vi "UHR-Fleezers Control (host) - 11.8.vi"() -> ()   [LabVIEW 2014] (continued)
                n1966 = property on="Sample Channel\nFlow" class="Bool (strict)"("Val(Sgnl)"=TRUE ("Value (Signaling)")) -> ()  [unwired: 2 in, 2 out]
              }
            }
          }
          frame #1 {
            n1967 = property on="Inject Pump 3" class="Bool (strict)"("Val(Sgnl)"=FALSE ("Value (Signaling)")) -> ()  [unwired: 2 in, 2 out]
            n1968 = local write "Target"(FALSE ("Target")) -> ()
          }
          frame #2 {
            n1969 = property on="Move Cap. 1 (DNA Bottom)" class="Bool (strict)"("Val(Sgnl)"=TRUE ("Value (Signaling)")) -> ()  [unwired: 2 in, 2 out]
          }
        }
      }
      event "Force FB Script": Value Change {
        n1970 = event-data() -> ()  [unwired: 1 in, 5 out]
        n1971 = local write "Force FB Script"(FALSE ("Force FB Data\nScript")) -> ()
        n1972 = flat-sequence {
          tunnel: w2821 -> [w2825]
          tunnel: w2822 -> [w2826]
          tunnel: [w2826] -> w2817
          tunnel: [w2825] -> w2816
          tunnel: w2817 -> [w2829]
          tunnel: w2816 -> [w2828]
          tunnel: ["Trap Trig Fl."] -> w2818
          tunnel: [w2871] -> w2819
          tunnel: w2818 -> [w2871]
          tunnel: [w2875] -> w2820
          tunnel: w2819 -> [w2875]
          tunnel: w2820 -> [w2877]
          frame #0 {
            n1973 = property on="Trap D (MHz)" class="DigNum (strict)"("Val(Sgnl)"="Trap D Before Moving") -> ()  [unwired: 2 in, 2 out]
          }
          frame #1 {
            n1974 = local read "Saved Stage Positions"() -> (w2831:dbl[][])
            n1975 = local write "FB Trap Pos Offset"(0.0 ("FB Trap Pos Offset")) -> ()
            n1976 = property on="Trap Pos. FB Offset Factor" class="DigNum (strict)"("Val(Sgnl)"=i64 0 ("Value (Signaling)")) -> ()  [unwired: 2 in, 2 out]
            n1977 = local write "Stage Moving"(TRUE ("Stage Moving")) -> ()
            n1978 = call "move to saved stage position.vi"("error in"=w2828, "Stage VISA resource name in"=w2829, "Position"="Stage Position To Establish FB", "Saved Stage Positions"=w2831) -> ("error out"=w2827:errorcluster)  [unwired: 1 out]
            n1979 = local write "Stage Control Serial Error"(w2827) -> ()
          }
          frame #2 {
            n1980 = call <vilib>:"Beep.vi"("duration (msec)"=u32 100, "frequency (Hz)"=u32 20) -> ()  [unwired: 1 in, 9 out]
            n1981 = local write "Stage Moving"(FALSE ("Stage Moving")) -> ()
            n1982 = property on="Tab Control 2" class="TabCtl (strict)"("Val(Sgnl)"=T6."Feedback on Trap Position" ("Value (Signaling)")) -> ()  [unwired: 2 in, 2 out]
            n1983 = stacked-sequence {
              frame #0 {
                n1984 = Multiply(x="Wait (s)", y=u32 1000 ("milliseconds to wait")) -> (x*y=w2840:u32)
                n1985 = property on="Trap D (MHz)" class="DigNum (strict)"("Val(Sgnl)"="Starting Trap D (MHz)") -> ()  [unwired: 2 in, 2 out]
                n1986 = Wait (ms)(milliseconds to wait=w2840) -> ()  [unwired: 1 out]
              }
              frame #1 {
                n1987 = property on="Set Reading to\nSetpoint" class="Bool (strict)"("Val(Sgnl)"=TRUE ("Value (Signaling)")) -> ()  [unwired: 2 in, 2 out]
              }
            }
            n1988 = property on="Tab Control" class="TabCtl (strict)"("Val(Sgnl)"=T4."Trap Control (RF)" ("Value (Signaling)")) -> ()  [unwired: 2 in, 2 out]
          }
          frame #3 {
            n1989 = Wait (ms)(milliseconds to wait=u32 500) -> ()  [unwired: 1 out]
          }
          frame #4 {
            n1990 = property on="Trap Pos. FB ON" class="Bool (strict)"("Val(Sgnl)"=TRUE ("Value (Signaling)")) -> ()  [unwired: 2 in, 2 out]
            n1991 = Wait (ms)(milliseconds to wait=u32 250) -> ()  [unwired: 1 out]
          }
          frame #5 {
            n1992 = case shown="\"0\", Default" "Remove Action Offset Dropdown" {
              tunnel: TRUE ("Value (Signaling)") -> [w2852 w2860 w2868]
              frame "1" {
                n1993 = flat-sequence {
                  tunnel: w2852 -> [w2859]
                  frame #0 {
                    n1994 = local read "factor"() -> (w2854:dbl)
                    n1995 = Greater Than 0?(x=w2854) -> (x > 0?=w2858:bool)
                    n1996 = Select(t=1.0, s=w2858, f=-1.0) -> (s? t:f=w2855:dbl)
                    n1997 = Multiply(x=w2855, y=w2854) -> (x*y=w2853:dbl)
                    n1998 = local write "factor"(w2853) -> ()
                  }
                  frame #1 {
                    n1999 = property on="Remove Offset to factor" class="Bool (strict)"("Val(Sgnl)"=w2859) -> ()  [unwired: 2 in, 2 out]
                  }
                }
              }
              frame "2" {
                n2000 = flat-sequence {
                  tunnel: w2860 -> [w2867]
                  frame #0 {
                    n2001 = local read "factor"() -> (w2861:dbl)
                    n2002 = Greater Than 0?(x=w2861) -> (x > 0?=w2866:bool)
                    n2003 = Select(t=-1.0, s=w2866, f=1.0) -> (s? t:f=w2864:dbl)
                    n2004 = Multiply(x=w2861, y=w2864) -> (x*y=w2863:dbl)
                    n2005 = local write "factor"(w2863) -> ()
                  }
                  frame #1 {
                    n2006 = property on="Remove Offset to factor" class="Bool (strict)"("Val(Sgnl)"=w2867) -> ()  [unwired: 2 in, 2 out]
                  }
                }
              }
              frame "0", Default {
                n2007 = property on="Remove Action Offset" class="Bool (strict)"("Val(Sgnl)"=w2868) -> ()  [unwired: 2 in, 2 out]
              }
            }
            n2008 = case shown="False" "Trap Trig Fl." {
              frame False {
                n2009 = case shown="True" "Green ON after FB ON?" {
                  selector: "Green ON after FB ON?" -> [_ w2870]
                  frame False {
                  }
                  frame True {
                    n2010 = property on="Green Laser ON/Interlacing" class="Bool (strict)"("Val(Sgnl)"=w2870) -> ()  [unwired: 2 in, 2 out]
                  }
                }
              }
              frame True {
              }
            }
            n2011 = Wait (ms)(milliseconds to wait=u32 250) -> ()  [unwired: 1 out]
          }
          frame #6 {
            n2012 = property on="Start Saving" class="Bool (strict)"("Val(Sgnl)"=TRUE ("Value (Signaling)")) -> ()  [unwired: 2 in, 2 out]
            n2013 = Wait (ms)(milliseconds to wait=u32 5000) -> ()  [unwired: 1 out]
          }
          frame #7 {
            w2874 = TRUE ("Value (Signaling)")
            n2014 = property on="Rem fb disp offset" class="Bool (strict)"("Val(Sgnl)"=w2874) -> ()  [unwired: 2 in, 2 out]
            n2015 = property on="Remove Offset" class="Bool (strict)"("Val(Sgnl)"=w2874) -> ()  [unwired: 2 in, 2 out]
            n2016 = Wait (ms)(milliseconds to wait=u32 100) -> ()  [unwired: 1 out]
          }
          frame #8 {
            n2017 = case shown="True" w2877 {
              frame False {
              }
              frame True {
                n2018 = local write "Trap Trig. Fl."(TRUE ("Value (Signaling)")) -> ()
              }
            }
          }
          frame #9 {
            n2019 = local read "Tether"() -> (w2880:bool)
            n2020 = And(x="Start dipping after?", y=w2880) -> (x .and. y?=w2879:bool)
            n2021 = case shown="True" w2879 {
              frame False {
              }
              frame True {
                n2022 = flat-sequence {
                  frame #0 {
                    n2023 = Multiply(x="Delay before dipping (s)", y=1000.0) -> (x*y=w2883:dbl)
                    n2024 = Wait (ms)(milliseconds to wait=w2883) -> ()  [unwired: 1 out]
                  }
                  frame #1 {
                    n2025 = property on="Dip for Protein" class="Bool (strict)"("Val(Sgnl)"=TRUE ("Value (Signaling)")) -> ()  [unwired: 2 in, 2 out]
                    n2026 = local write "Scripts"(T29."Dipping") -> ()
                  }
                }
              }
            }
          }
        }
      }
      event "Rupture Script": Value Change {
        n2027 = event-data() -> ()  [unwired: 1 in, 5 out]
        n2028 = local write "Rupture Script"(FALSE ("Rupture Script")) -> ()
        n2029 = flat-sequence {
          frame #0 {
            w2889 = TRUE
            w2894 = FALSE
            # "Number 6 for now is the\nrupture-experiment\nparameters."
            n2030 = local read "Starting Trap D (MHz)"() -> (w2895:dbl)
            n2031 = local write "Restart DMA? (AOD)"(w2894) -> ()
            n2032 = Replace Array Subset(array=u32[] [0] ("Index Values"), new element=6, index=0) -> (w2890:u32[])
            n2033 = local write "Save scans"(w2894) -> ()
            n2034 = property on="Trap D (MHz)" class="DigNum (strict)"("Val(Sgnl)"=w2895) -> ()  [unwired: 2 in, 2 out]
            n2035 = property on="Saved AOD Raster Scan Parameter Sets" class="Arr (strict)"("Index Values"=w2890) -> ()  [unwired: 2 in, 2 out]
            n2036 = property on="Start Saving" class="Bool (strict)"("Val(Sgnl)"=w2889) -> ()  [unwired: 2 in, 2 out]
            n2037 = property on="Green Laser ON/Interlacing" class="Bool (strict)"("Val(Sgnl)"=w2889) -> ()  [unwired: 2 in, 2 out]
          }
          frame #1 {
            n2038 = property on="Load parameters" class="Bool (strict)"("Val(Sgnl)"=TRUE ("Value (Signaling)")) -> ()  [unwired: 2 in, 2 out]
          }
        }
      }
      event "Fixed Traps Script": Value Change {
        n2039 = event-data() -> ()  [unwired: 1 in, 5 out]
        n2040 = local write "Fixed Traps Script"(FALSE ("Fixed Traps Data\nScript")) -> ()
        n2041 = flat-sequence {
          frame #0 {
            n2042 = case shown="True" "Green ON" {
              frame False {
              }
              frame True {
                n2043 = property on="Green Laser ON/Interlacing" class="Bool (strict)"("Val(Sgnl)"=TRUE) -> ()  [unwired: 2 in, 2 out]
              }
            }
            n2044 = local write "Offset (nm)"(0.0 ("Offset (nm)")) -> ()
            n2045 = property on="Sample Channel\nFlow" class="Bool (strict)"("Val(Sgnl)"=FALSE ("Value (Signaling)")) -> ()  [unwired: 2 in, 2 out]
            n2046 = property on="Trap D (MHz)" class="DigNum (strict)"("Val(Sgnl)"="Fixed Traps Trap Delta (MHz)") -> ()  [unwired: 2 in, 2 out]
          }
          frame #1 {
            n2047 = Wait (ms)(milliseconds to wait=u32 1000) -> ()  [unwired: 1 out]
          }
          frame #2 {
            n2048 = local write "Start Saving"(TRUE ("Start Saving")) -> ()
          }
          frame #3 {
            n2049 = local read "Bead Sep. Int. Time (s)"() -> (w2905:dbl)
            n2050 = Multiply(x=w2905, y=1000.0) -> (x*y=w2907:dbl)
            n2051 = Wait (ms)(milliseconds to wait=w2907) -> ()  [unwired: 1 out]
          }
          frame #4 {
            n2052 = property on="Remove Offset" class="Bool (strict)"("Val(Sgnl)"=TRUE ("Value (Signaling)")) -> ()  [unwired: 2 in, 2 out]
          }
          frame #5 {
            n2053 = property on="Dip for Protein" class="Bool (strict)"("Val(Sgnl)"="Start dipping after?") -> ()  [unwired: 2 in, 2 out]
          }
        }
      }
      event "Got DNA bead": Value Change {
        n2054 = event-data() -> ()  [unwired: 1 in, 5 out]
        n2055 = flat-sequence {
          frame #0 {
            n2056 = local read "Daq spot flow on"() -> (w2912:bool)
            n2057 = case shown="True" w2912 {
              frame False {
              }
              frame True {
                n2058 = property on="Sample Channel\nFlow" class="Bool (strict)"("Val(Sgnl)"=TRUE ("Value (Signaling)")) -> ()  [unwired: 2 in, 2 out]
              }
            }
            n2059 = property on="Got DNA bead" class="Bool"("Key Focus"=FALSE) -> ()  [unwired: 2 in, 2 out]
          }
          frame #1 {
            n2060 = property on="Inject Pump 1" class="Bool (strict)"("Val(Sgnl)"=FALSE ("Value (Signaling)")) -> ()  [unwired: 2 in, 2 out]
          }
          frame #2 {
            n2061 = property on="Cal/Data Acq. Spot" class="Bool (strict)"("Val(Sgnl)"=TRUE ("Value (Signaling)")) -> ()  [unwired: 2 in, 2 out]
          }
        }
      }
      event "Take Stepping Data": Value Change {
        n2062 = event-data() -> ()  [unwired: 1 in, 5 out]
        n2063 = local read "Save ave N"() -> (w2924:dbl)
        n2064 = flat-sequence {
          tunnel: w2924 -> [w2926]
          tunnel: [w2926] -> w2919
          tunnel: [w2928] -> w2920
          tunnel: w2919 -> [w2928]
          tunnel: [w2930] -> w2921
          tunnel: w2920 -> [w2930]
          tunnel: [w2933] -> w2922
          tunnel: w2921 -> [w2933]
          tunnel: [w2935] -> w2923
          tunnel: w2922 -> [w2935]
          tunnel: [w2937] -> w2917
          tunnel: w2923 -> [w2937]
          tunnel: w2917 -> [w2940]
          tunnel: [w2940] -> w2916
          tunnel: w2916 -> [w2941]
          tunnel: [w2941] -> w2918
          tunnel: w2918 -> [w2947]
          frame #0 {
            n2065 = property on="Save ave N" class="DigNum (strict)"("Val(Sgnl)"="Save ave factor") -> ()  [unwired: 2 in, 2 out]
          }
          frame #1 {
            n2066 = Wait (ms)(milliseconds to wait=u32 100) -> ()  [unwired: 1 out]
          }
          frame #2 {
            n2067 = local read "Offset 2 Start (MHz)"() -> (w2932:dbl)
            n2068 = property on="Saved AOD Raster Scan Parameter Sets" class="Arr (strict)"("Index Values"=u32[] [2]) -> ()  [unwired: 2 in, 2 out]
            n2069 = property on="Trap D (MHz)" class="DigNum (strict)"("Val(Sgnl)"=w2932) -> ()  [unwired: 2 in, 2 out]
          }
          frame #3 {
            n2070 = property on="Load parameters" class="Bool (strict)"("Val(Sgnl)"=TRUE ("Value (Signaling)")) -> ()  [unwired: 2 in, 2 out]
          }
          frame #4 {
            n2071 = Wait (ms)(milliseconds to wait=u32 100) -> ()  [unwired: 1 out]
          }
          frame #5 {
            n2072 = property on="Trap Raster Scan" class="Bool (strict)"("Val(Sgnl)"=TRUE ("Value (Signaling)")) -> ()  [unwired: 2 in, 2 out]
          }
          frame #6 {
            n2073 = Wait (ms)(milliseconds to wait=u32 1000) -> ()  [unwired: 1 out]
          }
          frame #7 {
            n2074 = while {
              stop <- w2944 stop-if-true
              n2075 = local read "Raster Scanning..."() -> (w2946:bool)
              n2076 = local read "Saving..."() -> (w2945:bool)
              n2077 = Not(x=w2945) -> (.not. x?=w2942:bool)
              n2078 = Not(x=w2946) -> (.not. x?=w2943:bool)
              n2079 = And(x=w2943, y=w2942) -> (x .and. y?=w2944:bool)
            }
          }
          frame #8 {
            n2080 = property on="Save ave N" class="DigNum (strict)"("Val(Sgnl)"=w2947) -> ()  [unwired: 2 in, 2 out]
          }
        }
      }
      event "Step Size (nm)": Value Change {
        n2081 = event-data() -> ()  [unwired: 1 in, 5 out]
        n2082 = flat-sequence {
          frame #0 {
            n2083 = property on="Saved AOD Raster Scan Parameter Sets" class="Arr (strict)"("Index Values"=u32[] [1]) -> ()  [unwired: 2 in, 2 out]
          }
          frame #1 {
            n2084 = Multiply(x="N Steps", y="Step Size (nm)") -> (x*y=w2949:dbl)
            n2085 = property on="Scan Speed AOD (nm/s) 2" class="DigNum (strict)"("Value"="Step Size (nm)") -> ()  [unwired: 2 in, 2 out]
            n2086 = property on="Step Size AOD (nm) 2" class="DigNum (strict)"("Value"="Step Size (nm)") -> ()  [unwired: 2 in, 2 out]
            n2087 = property on="Scan Range AOD (nm) 2" class="DigNum (strict)"("Value"=w2949) -> ()  [unwired: 2 in, 2 out]
          }
        }
      }
      event "Take Detection Laser\nImage": Value Change {
        n2088 = event-data() -> ()  [unwired: 1 in, 5 out]
        n2089 = flat-sequence {
          tunnel: [w2977] -> w2967
          tunnel: [w2976] -> w2960
          tunnel: [w2975] -> w2952
          tunnel: [w2980] -> w2968
          tunnel: w2967 -> [w2980]
          tunnel: [w2979] -> w2961
          tunnel: w2960 -> [w2979]
          tunnel: [w2978] -> w2953
          tunnel: w2952 -> [w2978]
          tunnel: [w2984] -> w2969
          tunnel: w2968 -> [w2984]
          tunnel: [w2983] -> w2962
          tunnel: w2961 -> [w2983]
          tunnel: [w2982] -> w2954
          tunnel: w2953 -> [w2982]
          tunnel: [w2990] -> w2970
          tunnel: w2969 -> [w2990]
          tunnel: [w2989] -> w2963
          tunnel: w2962 -> [w2989]
          tunnel: [w2988] -> w2955
          tunnel: w2954 -> [w2988]
          tunnel: [w2994] -> w2971
          tunnel: w2970 -> [w2994]
          tunnel: [w2993] -> w2964
          tunnel: w2963 -> [w2993]
          tunnel: [w2992] -> w2956
          tunnel: w2955 -> [w2992]
          tunnel: [w2998] -> w2972
          tunnel: w2971 -> [w2998]
          tunnel: [w2997] -> w2965
          tunnel: w2964 -> [w2997]
          tunnel: [w2996] -> w2957
          tunnel: w2956 -> [w2996]
          tunnel: [w3002] -> w2973
          tunnel: w2972 -> [w3002]
          tunnel: [w3001] -> w2966
          tunnel: w2965 -> [w3001]
          tunnel: [w3000] -> w2958
          tunnel: w2957 -> [w3000]
          tunnel: w2973 -> [w3008]
          tunnel: w2966 -> [w3007]
          tunnel: [w3005] -> w2959
          tunnel: w2958 -> [w3005]
          tunnel: w2959 -> [w3009]
          frame #0 {
            n2090 = local read "Green Laser ON/Interlacing"() -> (w2977:bool)
            n2091 = local read "Green laser mode"() -> (w2976:enum32{"Laser ON", "Laser OFF", "Interlace"})
            n2092 = local read "Green FB On/Off"() -> (w2975:bool)
          }
          frame #1 {
            n2093 = property on="Green FB On/Off" class="Bool (strict)"("Val(Sgnl)"=FALSE ("Value (Signaling)")) -> ()  [unwired: 2 in, 2 out]
          }
          frame #2 {
            n2094 = property on="Green Laser ON/Interlacing" class="Bool (strict)"("Val(Sgnl)"=TRUE ("Value (Signaling)")) -> ()  [unwired: 2 in, 2 out]
            n2095 = property on="Flip Green Filter" class="Bool (strict)"("Val(Sgnl)"=TRUE ("Value (Signaling)")) -> ()  [unwired: 2 in, 2 out]
            n2096 = property on="Green laser mode" class="RadioBtnsControl (strict)"("Val(Sgnl)"=enum32{"Laser ON", "Laser OFF", "Interlace"}."Laser ON" ("Value (Signaling)")) -> ()  [unwired: 2 in, 2 out]
          }
          frame #3 {
            n2097 = Wait (ms)(milliseconds to wait=u32 500) -> ()  [unwired: 1 out]
          }
          frame #4 {
            n2098 = property on="Confocal\nImage" class="Bool (strict)"("Val(Sgnl)"=TRUE ("Value (Signaling)")) -> ()  [unwired: 2 in, 2 out]
          }
          frame #5 {
            n2099 = Wait (ms)(milliseconds to wait=u32 2000) -> ()  [unwired: 1 out]
          }
          frame #6 {
            n2100 = while {
              stop <- w3003 stop-if-true
              n2101 = local read "Saving..."() -> (w3004:bool)
              n2102 = Not(x=w3004) -> (.not. x?=w3003:bool)
            }
          }
          frame #7 {
            n2103 = property on="Flip Green Filter" class="Bool (strict)"("Val(Sgnl)"=TRUE ("Value (Signaling)")) -> ()  [unwired: 2 in, 2 out]
            n2104 = property on="Green Laser ON/Interlacing" class="Bool (strict)"("Val(Sgnl)"=w3008) -> ()  [unwired: 2 in, 2 out]
            n2105 = property on="Green laser mode" class="RadioBtnsControl (strict)"("Val(Sgnl)"=w3007) -> ()  [unwired: 2 in, 2 out]
          }
          frame #8 {
            n2106 = property on="Green FB On/Off" class="Bool (strict)"("Val(Sgnl)"=w3009) -> ()  [unwired: 2 in, 2 out]
          }
        }
      }
      event "Stop All": Value Change {
        n2107 = event-data() -> ()  [unwired: 1 in, 5 out]
        n2108 = local read "Stop All"() -> (w3010:bool)
      }
    }
    n2109 = node-c288() -> ()  [unwired: 1 in, 1 out]
  }
  n2110 = timed-loop "Mouse control: trap position (AOM deflection), set confocal spot from image" {
    tunnel: [w3012] -> w198
    tunnel: w18 -> [w3011]
    timing: w110 -> [_]
    timing-out: [_] -> w109
    stop <- w3012 stop-if-true
    n2111 = node-c288() -> ()  [unwired: 2 out]
    n2112 = event shown="[0] \"Pane\": Mouse Down" {
      selector: _ -> [_ _]
      dyn-events: _ -> [_ _]
      timeout: _ -> [_ _]
      tunnel: w3011 -> [w3015 _]
      event Mouse Down {
        n2113 = event-data() -> ("Time"=w3017:u32, "Coords"=w3016:T7, "Button"=w3018:u16)  [unwired: 6 out]
        n2114 = case shown="3" w3018 {
          tunnel: w3017 -> [_ _ w3157]
          tunnel: w3016 -> [_ w3023 w3155]
          tunnel: w3015 -> [_ _ w3153]
          frame 0, Default {
          }
          frame 1 {
            n2115 = property on="APD 2" class="ImageControl"() -> ("Displayed Image Position"=w3037:cluster{"Left":i32, "Top":i32})  [unwired: 2 in, 2 out]
            n2116 = control-ref of="Primary Video Display"() -> (w3030:refnum<vi>)
            n2117 = property on="APD 1" class="ImageControl"() -> ("Displayed Image Position"=w3066:cluster{"Left":i32, "Top":i32})  [unwired: 2 in, 2 out]
            n2118 = property on="Detection Laser X" class="ImageControl"() -> ("Displayed Image Position"=w3063:cluster{"Left":i32, "Top":i32})  [unwired: 2 in, 2 out]
            n2119 = property on="Detection Laser Y" class="ImageControl"() -> ("Displayed Image Position"=w3062:cluster{"Left":i32, "Top":i32})  [unwired: 2 in, 2 out]
            n2120 = property on="APD 2" class="ImageControl"() -> ("Displayed Image Size"=w3036:cluster{"Width":u32, "Height":u32})  [unwired: 2 in, 2 out]
            n2121 = property on="APD 1" class="ImageControl"() -> ("Displayed Image Size"=w3064:cluster{"Width":u32, "Height":u32})  [unwired: 2 in, 2 out]
            n2122 = property on="Detection Laser X" class="ImageControl"() -> ("Displayed Image Size"=w3065:cluster{"Width":u32, "Height":u32})  [unwired: 2 in, 2 out]
            n2123 = property on="Detection Laser Y" class="ImageControl"() -> ("Displayed Image Size"=w3061:cluster{"Width":u32, "Height":u32})  [unwired: 2 in, 2 out]
            n2124 = property class="ImageControl"(reference=w3030) -> ("Displayed Image Position"=w3028:cluster{"Left":i32, "Top":i32})  [unwired: 1 in, 2 out]
            n2125 = property class="ImageControl"(reference=w3030) -> ("Displayed Image Size"=w3029:cluster{"Width":u32, "Height":u32})  [unwired: 1 in, 2 out]
            n2126 = Unbundle By Name(w3036) -> ("Width"=w3033:u32, "Height"=w3032:u32)
            n2127 = Unbundle By Name(w3037) -> ("Left"=w3035:i32, "Top"=w3034:i32)
            n2128 = Unbundle By Name(w3064) -> ("Width"=w3058:u32, "Height"=w3057:u32)
            n2129 = Unbundle By Name(w3065) -> ("Width"=w3054:u32, "Height"=w3053:u32)
            n2130 = Unbundle By Name(w3061) -> ("Width"=w3050:u32, "Height"=w3049:u32)
            n2131 = Unbundle By Name(w3066) -> ("Left"=w3060:i32, "Top"=w3059:i32)
            n2132 = Unbundle By Name(w3063) -> ("Left"=w3056:i32, "Top"=w3055:i32)
            n2133 = Unbundle By Name(w3062) -> ("Left"=w3052:i32, "Top"=w3051:i32)
            n2134 = Bundle("Left"=w3035, "Top"=w3034, "Width"=w3033, "Height"=w3032) -> (w3031:T30)  [unwired: 1 in]
            n2135 = Bundle("Left"=w3060, "Top"=w3059, "Width"=w3058, "Height"=w3057) -> (w3048:T30)  [unwired: 1 in]
            n2136 = Bundle("Left"=w3056, "Top"=w3055, "Width"=w3054, "Height"=w3053) -> (w3047:T30)  [unwired: 1 in]
            n2137 = Bundle("Left"=w3052, "Top"=w3051, "Width"=w3050, "Height"=w3049) -> (w3046:T30)  [unwired: 1 in]
            n2138 = Unbundle By Name(w3029) -> ("Width"=w3025:u32, "Height"=w3024:u32)
            n2139 = Unbundle By Name(w3028) -> ("Left"=w3027:i32, "Top"=w3026:i32)
            n2140 = Build Cluster Array(w3031, w3048, w3047, w3046) -> (w3045:T31)
            n2141 = Bundle("Left"=w3027, "Top"=w3026, "Width"=w3025, "Height"=w3024) -> (w3020:T30)  [unwired: 1 in]
            n2142 = for {
              tunnel: w3023 -> [w3099]
              tunnel: w3045 -> [w3100] mode=indexing
              shift-right: [w3097] -> w3043
              shift-left: TRUE -> [w3098]
              shift-right: [w3096] -> w3041
              shift-left: _ -> [w3092]
              shift-right: [w3095] -> w3040
              shift-left: _ -> [w3091]
              shift-right: [w3094] -> w3039
              shift-left: _ -> [w3090]
              shift-right: [w3093] -> w3038
              shift-left: _ -> [w3089]
              n2143 = case shown="True" w3098 {
                selector: w3098 -> [w3105 _]
                tunnel: w3100 -> [_ w3114]
                tunnel: w3099 -> [_ w3112]
                tunnel: [w3105 w3110] -> w3097
                tunnel: [w3104 w3109] -> w3096
                tunnel: [w3103 w3108] -> w3095
                tunnel: [w3102 w3107] -> w3094
                tunnel: [w3101 w3106] -> w3093
                tunnel: w3092 -> [w3104 _]
                tunnel: w3091 -> [w3103 _]
                tunnel: w3090 -> [w3102 _]
                tunnel: w3089 -> [w3101 _]
                frame False {
                }
                frame True {
                  n2144 = Unbundle(w3114) -> (w3113:T30)
                  n2145 = call "isclickinwindow.vi"("Image Param"=w3113, "Point32"=w3112) -> ("4 Y"=w3106:i32, "3 Height"=w3107:i32, "2 X"=w3108:i32, "1 Width"=w3109:i32, "In image?"=w3111:bool)  [unwired: 1 in]
                  n2146 = Not(x=w3111) -> (.not. x?=w3110:bool)
                }
              }
            }
            n2147 = call "isclickinwindow.vi"("Image Param"=w3020, "Point32"=w3023) -> ("4 Y"=w3021:i32, "2 X"=w3022:i32, "In image?"=w3019:bool)  [unwired: 1 in, 2 out]
            n2148 = case shown="True" w3019 {
              tunnel: w3022 -> [_ w3070]
              tunnel: w3021 -> [_ w3073]
              frame False {
              }
              frame True {
                w3082 = 2
                n2149 = Subtract(x=480, y=w3073) -> (x-y=w3072:i32)
                n2150 = Unbundle("Target size") -> ("Width"=w3083:dbl, "Height"=w3081:dbl)
                n2151 = Subtract(x=w3070, y=2) -> (x-y=w3069:i32)
                n2152 = Divide(x=w3081, y=w3082) -> (x/y=w3079:dbl)
                n2153 = Divide(x=w3083, y=w3082) -> (x/y=w3080:dbl)
                n2154 = Subtract(x=w3069, y=w3080) -> (x-y=w3078:dbl)
                n2155 = Add(x=w3069, y=w3080) -> (x+y=w3076:dbl)
                n2156 = Subtract(x=w3072, y=w3079) -> (x-y=w3077:dbl)
                n2157 = Add(x=w3072, y=w3079) -> (x+y=w3075:dbl)
                n2158 = Bundle(w3069, w3072) -> (w3085:cluster{i32, i32})  [unwired: 1 in]
                n2159 = Bundle(w3078, w3077, w3076, w3075) -> (w3067:cluster{dbl, dbl, dbl, dbl})  [unwired: 1 in]
                n2160 = case shown="True" "Set target" {
                  tunnel: w3085 -> [_ w3088]
                  tunnel: w3067 -> [_ w3086]
                  frame False {
                  }
                  frame True {
                    n2161 = local write "Target coordinates"(w3086) -> ()
                    n2162 = local write "Set target"(FALSE ("Set target")) -> ()
                    "Video coordinates" <- w3088
                  }
                }
              }
            }
            n2163 = Not(x=w3043) -> (.not. x?=w3042:bool)
            n2164 = case shown="True" w3042 {
              tunnel: w3040 -> [_ w3128]
              tunnel: w3038 -> [_ w3127]
              tunnel: w3041 -> [_ w3126]
              tunnel: w3039 -> [_ w3125]
              frame False {
              }
              frame True {
                w3115 = FALSE ("Get Point")
                n2165 = local read "Scan lines (y)"() -> (w3130:u64)
                n2166 = disable-structure shown="Disabled" {
                  frame Disabled {
                  }
                  frame Enabled {
                  }
                }
                n2167 = local read "Actual MCL Inc (V)"() -> (w3124:dbl)
                n2168 = local read "Scan steps (MCL)"() -> (w3129:u64)
                n2169 = Divide "Y Pix/step"(x=w3125, y=w3130) -> (x/y=w3137:dbl)
                n2170 = Divide "Y V/pix"(x=w3124, y=w3137) -> (x/y=w3136:dbl)
                n2171 = Divide "Y half step offset"(x=w3124, y=2.0) -> (x/y=w3138:dbl)
                n2172 = Divide "X pix/step"(x=w3126, y=w3129) -> (x/y=w3135:dbl)
                n2173 = Negate(x=w3138) -> (-x=w3139:dbl)
                n2174 = local read "Initial Y"() -> (w3145:dbl)
                n2175 = Multiply(x=w3127, y=w3136) -> (x*y=w3146:dbl)
                n2176 = Divide "X half step offset"(x=w3124, y=2.0) -> (x/y=w3132:dbl)
                n2177 = Divide "X V/pix"(x=w3124, y=w3135) -> (x/y=w3134:dbl)
                n2178 = Multiply(x=w3124, y=w3129) -> (x*y=w3141:dbl)
                n2179 = Compound Arithmetic op=ADD(w3139, w3146, w3145) -> (w3116:dbl)
                "Pointer Y (V)" <- w3116
                n2180 = Multiply(x=w3134, y=w3128) -> (x*y=w3143:dbl)
                n2181 = Negate(x=w3132) -> (-x=w3131:dbl)
                n2182 = local read "Initial X"() -> (w3144:dbl)
                n2183 = Negate(x=w3143) -> (-x=w3142:dbl)
                n2184 = Compound Arithmetic op=ADD(w3131, w3141, w3144, w3142) -> (w3117:dbl)
                "Pointer X (V)" <- w3117
                n2185 = case shown="True" "Set High F Confocal Spot (X-Y)" {
                  tunnel: w3117 -> [_ w3147]
                  tunnel: w3116 -> [_ w3148]
                  frame False {
                  }
                  frame True {
                    "Confocal Y 2 (V)" <- w3148
                    "Confocal X 2 (V)" <- w3147
                  }
                }
                n2186 = Or(x="Set X Only", y="Set Confocal Spot (X-Y)") -> (x .or. y?=w3120:bool)
                n2187 = Or(x="Set Confocal Spot (X-Y)", y="Set Y Only") -> (x .or. y?=w3119:bool)
                n2188 = case shown="True" w3120 {
                  tunnel: w3117 -> [_ w3149]
                  frame False {
                  }
                  frame True {
                    n2189 = property on="AO2" class="Slide (strict)"("Val(Sgnl)"=w3149) -> ()  [unwired: 2 in, 2 out]
                    "Confocal X 1 (V)" <- w3149
                  }
                }
                n2190 = case shown="True" w3119 {
                  tunnel: w3116 -> [_ w3150]
                  frame False {
                  }
                  frame True {
                    n2191 = property on="AO1" class="Slide (strict)"("Val(Sgnl)"=w3150) -> ()  [unwired: 2 in, 2 out]
                    "Confocal Y 1 (V)" <- w3150
                  }
                }
                n2192 = local write "Set High F Confocal Spot (X-Y)"(w3115) -> ()
                n2193 = local write "Set Confocal Spot (X-Y)"(w3115) -> ()
                n2194 = local write "Set X Only"(w3115) -> ()
                n2195 = local write "Set Y Only"(w3115) -> ()
              }
            }
          }
          frame 3 {
            n2196 = local read "BD 2 Frequency 1 (MHz)"() -> (w3151:dbl)
            n2197 = local read "BD 1 Frequency 1 (MHz)"() -> (w3152:dbl)
            n2198 = local write "Manipulating Trap"(TRUE ("Manipulating Trap")) -> ()
            n2199 = local write "Coords"(T7 {"Horizontal"=0, "Vertical"=0} ("Coords")) -> ()
            n2200 = while {
              tunnel: w3157 -> [w3162]
              tunnel: w3155 -> [w3161]
              tunnel: w3153 -> [w3160]
              tunnel: w3152 -> [w3159]
              tunnel: w3151 -> [w3158]
              stop <- w3163 stop-if-true
              n2201 = event shown="[0] \"Pane\": Mouse Move" {
                selector: _ -> [_ _]
                dyn-events: _ -> [_ _]
                timeout: _ -> [_ _]
                tunnel: ["Force Manip Abort" w3227] -> w3163
                tunnel: w3162 -> [w3170 _]
                tunnel: w3161 -> [w3168 _]
                tunnel: w3160 -> [w3167 _]
                tunnel: w3159 -> [w3166 _]
                tunnel: w3158 -> [w3165 _]
                event Mouse Move {
                  n2202 = event-data() -> ("Time"=w3171:u32, "Coords"=w3172:T7)  [unwired: 3 out]
                  n2203 = Less?(x=w3171, y=w3170) -> (x < y?=w3169:bool)
                  n2204 = case "Makes sure old motion events prior to mouse click aren't used" shown="False" w3169 {
                    tunnel: w3172 -> [w3214 _]
                    tunnel: w3168 -> [w3215 _]
                    tunnel: w3167 -> [w3192 _]
                    tunnel: w3166 -> [w3188 _]
                    tunnel: w3165 -> [w3187 _]
                    frame False {
                      n2205 = Subtract(x=w3214, y=w3215) -> (x-y=w3213:T7)
                      "Coords" <- w3213
                      n2206 = local read "Y RF Frequency Limits (MHz)"() -> (w3173:T16)
                      n2207 = To Double Precision Float(number=w3213) -> (double precision float=w3212:cluster{"Horizontal":dbl, "Vertical":dbl})
                      n2208 = Multiply(x=cluster{"Horizontal":dbl, "Vertical":dbl} {"Horizontal"=-1.0, "Vertical"=1.0}, y="Manipulation Scaling") -> (x*y=w3208:cluster{"Horizontal":dbl, "Vertical":dbl})
                      n2209 = local read "X RF Frequency Limits (MHz)"() -> (w3174:T16)
                      n2210 = Multiply(x=w3212, y=w3208) -> (x*y=w3210:cluster{"Horizontal":dbl, "Vertical":dbl})
                      n2211 = Unbundle By Name(w3210) -> ("Horizontal"=w3205:dbl, "Vertical"=w3209:dbl)
                      n2212 = Unbundle By Name(w3173) -> ("Maximum"=w3176:dbl, "Minimum"=w3175:dbl)
                      n2213 = Boolean To (0,1)(Boolean="Manip. X?") -> (0, 1=w3203:i16)
                      n2214 = Boolean To (0,1)(Boolean="Manip. Y?") -> (0, 1=w3200:i16)
                      n2215 = local read "BD 1 Frequency 2 (MHz)"() -> (w3190:dbl)
                      n2216 = Multiply(x=w3209, y=w3200) -> (x*y=w3202:dbl)
                      n2217 = Multiply(x=w3203, y=w3205) -> (x*y=w3206:dbl)
                      n2218 = local read "BD 2 Frequency 2 (MHz)"() -> (w3189:dbl)
                      n2219 = Unbundle By Name(w3174) -> ("Maximum"=w3178:dbl, "Minimum"=w3177:dbl)
                      n2220 = Add(x=w3187, y=w3202) -> (x+y=w3180:dbl)
                      n2221 = Add(x=w3188, y=w3206) -> (x+y=w3182:dbl)
                      n2222 = In Range and Coerce(upper limit=w3178, x=w3182, lower limit=w3177) -> (coerced(x)=w3181:dbl)  [unwired: 1 out]
                      n2223 = In Range and Coerce(upper limit=w3176, x=w3180, lower limit=w3175) -> (coerced(x)=w3179:dbl)  [unwired: 1 out]
                      n2224 = Subtract(x=w3181, y=w3190) -> (x-y=w3199:dbl)
                      n2225 = Subtract(x=w3179, y=w3189) -> (x-y=w3198:dbl)
                      n2226 = Square(x=w3199) -> (x^2=w3197:dbl)
                      n2227 = Square(x=w3198) -> (x^2=w3196:dbl)
                      n2228 = Add(x=w3197, y=w3196) -> (x+y=w3195:dbl)
                      n2229 = Square Root(x=w3195) -> (sqrt(x)=w3191:dbl)
                      n2230 = In Range and Coerce(upper limit="Limit Max (MHz)", x=w3191, lower limit="Limit Min (MHz)") -> (In Range?=w3184:bool)  [unwired: 1 out]
                      n2231 = Not(x="Limits Enable") -> (.not. x?=w3183:bool)
                      n2232 = Or(x=w3184, y=w3183) -> (x .or. y?=w3185:bool)
                      n2233 = case shown="True" w3185 {
                        tunnel: w3192 -> [_ w3225]
                        tunnel: w3191 -> [_ w3216]
                        tunnel: w3181 -> [_ w3223]
                        tunnel: w3190 -> [_ w3222]
                        tunnel: w3179 -> [_ w3221]
                        tunnel: w3189 -> [_ w3220]
                        tunnel: w3174 -> [_ w3218]
                        tunnel: w3173 -> [_ w3217]
                        frame False {
                        }
                        frame True {
                          n2234 = local read "BD 1 Frequency 3 (MHz)"() -> (w3224:dbl)
                          n2235 = local read "BD 2 Frequency 3 (MHz)"() -> (w3219:dbl)
                          n2236 = local write "Trap D (MHz)"(w3216) -> ()
                          n2237 = call "set RF board frequency - interlace.vi"("Board 2 Frequency Limits"=w3217, "Board 1 Frequency Limits"=w3218, "FPGA VI Reference In"=w3225, "Board 2 Frequency 3 (MHz)"=w3219, "Board 1 Frequency 3 (MHz)"=w3224, "Board 2 Frequency 2 (MHz)"=w3220, "Board 2 Frequency 1 (MHz)"=w3221, "Board 1 Frequency 2 (MHz)"=w3222, "Board 1 Frequency 1  (MHz)"=w3223) -> ()  [unwired: 1 in, 2 out]
                          n2238 = local write "BD 2 Frequency 1 (MHz)"(w3221) -> ()
                          n2239 = local write "BD 1 Frequency 1 (MHz)"(w3223) -> ()
                        }
                      }
                    }
                    frame True {
                    }
                  }
                }
                event Mouse Up {
                  n2240 = event-data() -> ("Button"=w3226:u16)  [unwired: 8 out]
                  n2241 = case shown="3" w3226 {
                    tunnel: [FALSE TRUE] -> w3227
                    frame 0, Default {
                    }
                    frame 3 {
                      n2242 = local read "Trap D (MHz)"() -> (w3229:dbl)
                      n2243 = property on="Initial D (MHz)" class="DigNum (strict)"("Val(Sgnl)"=w3229) -> ()  [unwired: 2 in, 2 out]
                      n2244 = local write "Manipulating Trap"(FALSE ("Manipulating Trap")) -> ()
                    }
                  }
                }
              }
            }
          }
        }
      }
      event Mouse Move {
        n2245 = event-data() -> ()  [unwired: 6 out]
      }
    }
    n2246 = local read "Stop All"() -> (w3012:bool)
    n2247 = node-c288() -> ()  [unwired: 2 out]
  }
  n2248 = node-c288(w107) -> ()  [unwired: 1 out]
  n2249 = node-c288(w109) -> ()  [unwired: 1 out]
  n2250 = node-c288(w95) -> ()  [unwired: 1 out]
  n2251 = flat-sequence "Video" {
    tunnel: [w3240] -> w97
    tunnel: w97 -> [w3281]
    frame #0 {
      n2252 = while {
        stop <- w3233 continue-if-true
        n2253 = call "Close Video Capture.vi"() -> ("error code OUT"=w3235:i32)
        n2254 = Equal?(x=w3235, y=0) -> (x = y?=w3233:bool)
      }
      n2255 = local write "Stop All"(FALSE ("Stop All")) -> ()
    }
    frame #1 {
      n2256 = call "DMR_Init.vi"() -> ()  [unwired: 3 out]
    }
    frame #2 {
      # "Setting the destination format to Mono8 makes sure that the image can be displayed in the intensity plot."
      n2257 = call "DMR_GetDevice.vi"("search string IN"="DE019116701") -> ("device handle OUT"=w3258:i32)  [unwired: 4 in, 2 out]
      n2258 = call "DMR_OpenDevice.vi"("device handle IN"=w3258) -> ("driver handle OUT"=w3241:i32)  [unwired: 4 out]
      n2259 = call "DMR_FindList.vi"("flags IN"=u32 0 ("flags"), "list name IN"="" ("String"), "list type IN"=T32."camera descriptions", "driver handle IN"=w3241) -> ("list handle OUT"=w3244:i32)  [unwired: 2 out]
      n2260 = call "DMR_FindList.vi"("flags IN"=u32 0 ("flags"), "list name IN"="Base", "list type IN"=T32."setting", "driver handle IN"=w3241) -> ("list handle OUT"=w3242:i32)  [unwired: 2 out]
      n2261 = call "OBJ_GetHandle.vi"("object name IN"="VideoStandard", "list handle IN"=w3244) -> ("object handle OUT"=w3238:i32)  [unwired: 3 out]
      n2262 = call "OBJ_GetHandle.vi"("object name IN"="PixelFormat", "list handle IN"=w3242) -> ("object handle OUT"=w3252:i32)  [unwired: 3 out]
      n2263 = call "OBJ_SetS.vi"("value index IN"=0, "value IN"="NTSC M", "object handle IN"=w3238) -> ()  [unwired: 2 out]
      n2264 = call "OBJ_SetS.vi"("value index IN"=0, "value IN"="Mono8" ("value"), "object handle IN"=w3252) -> ()  [unwired: 2 out]
      n2265 = call "OBJ_GetHandle.vi"("object name IN"="VideoChannel", "list handle IN"=w3242) -> ("object handle OUT"=w3248:i32)  [unwired: 3 out]
      n2266 = while {
        tunnel: [w3263] -> w3240
        tunnel: w3241 -> [w3260]
        stop <- w3261 continue-if-true
        n2267 = call "DMR_ImageRequestSingle.vi"("request control IN"=0, "driver handle IN"=w3260) -> ("error code OUT"=w3262:i32, "driver handle OUT"=w3263:i32)  [unwired: 2 out]
        n2268 = Equal To 0?(x=w3262) -> (x = 0?=w3261:bool)
      }
      n2269 = call "OBJ_SetI.vi"("value index IN"=0, "value IN"=3 ("Video channel"), "object handle IN"=w3248) -> ()  [unwired: 2 out]
    }
    frame #3 {
      w3269 = T17 0 items=["Grayscale (U8)", "Grayscale (I16)", "Grayscale (SGL)", "Complex (CSG)", "RGB (U32)", "HSL (U32)", "RGB (U64)"] ("Image Type")
      w3277 = T17 0 items=["Grayscale (U8)", "Grayscale (I16)", "Grayscale (SGL)", "Complex (CSG)", "RGB (U32)", "HSL (U32)", "RGB (U64)"] ("Image Type")
      n2270 = for "Create Greyscale map" {
        N: 256 -> [_]
        tunnel: [w3283] -> w3266 mode=indexing
        workers-P: _ -> [_]
        i -> [w3286]
        n2271 = To Unsigned Byte Integer(number=w3286) -> (unsigned 8bit integer=w3282:u8)
        n2272 = Join Numbers(hi=w3282, lo=w3282) -> ((hi.lo)=w3285:u16)
        n2273 = Join Numbers(hi=w3282, lo=w3282) -> ((hi.lo)=w3284:u16)
        n2274 = Join Numbers(hi=w3285, lo=w3284) -> ((hi.lo)=w3283:u32)
      }
      n2275 = call "IMAQ Create"("Image Name"="Scaled video", "Image Type"=w3269) -> ("New Image"=w3268:T2)  [unwired: 2 in, 2 out]
      n2276 = call "IMAQ Create"("Image Name"="Main video", "Image Type"=w3277) -> ("New Image"=w3278:T2)  [unwired: 2 in, 2 out]
      n2277 = node-c288(0 ("Processor")) -> (w3276:T21)  [unwired: 3 out]
      n2278 = Initialize Array(u32 0 ("Window Number (0...15)"), 480 ("dimension size"), 640 ("dimension size")) -> (w3271:u32[][])
      n2279 = timed-loop {
        tunnel: w3281 -> [w3303]
        tunnel: [w3302] -> w3280
        tunnel: w3278 -> [w3301]
        timing: w3276 -> [_]
        timing-out: [_] -> w3275
        tunnel: w3271 -> [w3290]
        tunnel: w3268 -> [w3288]
        tunnel: w3266 -> [w3287]
        stop <- w3289 stop-if-true
        # "This block performs the \nactual image capture."
        n2280 = node-c288() -> ()  [unwired: 2 out]
        n2281 = local read "Stop All"() -> (w3289:bool)
        n2282 = Reciprocal(x="Video Capture Rate (Hz)") -> (1/x=w3293:dbl)
        n2283 = Multiply(x=w3293, y=1000.0) -> (x*y=w3291:dbl)
        n2284 = call "DMR_ImageRequestWaitFor.vi"("queue number IN"=0, "timeout(ms) IN"=500, "driver handle IN"=w3303) -> ("error code OUT"=w3307:i32, "request number OUT"=w3304:i32, "driver handle OUT"=w3305:i32)
        n2285 = feedback #1(T33 refnum ("Avi Refnum")) -> (w3295:T33)
        n2286 = case shown="True" "New Video File" {
          tunnel: [T33 refnum ("Avi Refnum") w3324] -> w3297
          tunnel: [FALSE TRUE] -> w3298
          tunnel: w3295 -> [_ w3320]
          frame False {
          }
          frame True {
            n2287 = call "Create new save file.vi"("Ext"=".avi" ("string"), "Index In"="Video Index") -> ("Path Out"=w3316:path, "Index Out"=w3317:dbl)  [unwired: 1 in]
            "Path Out" <- w3316
            n2288 = Not Equal?(x=w3320, y=T33 refnum ("Avi Refnum")) -> (x != y?=w3321:bool)
            n2289 = Increment(x=w3317) -> (x+1=w3326:dbl)
            n2290 = case shown="True" w3321 {
              tunnel: w3320 -> [_ w3327]
              frame False {
              }
              frame True {
                n2291 = call "IMAQ AVI Close"("Avi Refnum"=w3327) -> ()  [unwired: 1 in, 10 out]
              }
            }
            n2292 = local write "Video Index"(w3326) -> ()
            n2293 = call "IMAQ AVI Create"("Frames Per Second"=u32 30, "AVI Path"=w3316) -> ("Avi Refnum"=w3324:T33)  [unwired: 5 in, 4 out]
          }
        }
        n2294 = Equal To 0?(x=w3307) -> (x = 0?=w3306:bool)
        n2295 = Select(t=w3297, s=w3298, f=w3295) -> (s? t:f=w3296:T33)
        n2296 = feedback-in #1(w3296) -> ()
        n2297 = case shown="True" w3306 {
          tunnel: w3305 -> [w3328 w3355]
          tunnel: w3304 -> [_ w3354]
          tunnel: [w3328 w3351] -> w3302
          tunnel: w3301 -> [_ w3332]
          tunnel: w3290 -> [_ w3339]
          tunnel: w3296 -> [_ w3337]
          tunnel: w3288 -> [_ w3333]
          tunnel: w3287 -> [_ w3334]
          frame False {
          }
          frame True {
            w3345 = u32 0 ("X-offset IN")
            n2298 = call "DMR_GetImageRequestBufferData.vi"("driver handle IN"=w3355, "request number IN"=w3354) -> ("width OUT"=w3344:i32, "height OUT"=w3343:i32, "driver handle OUT"=w3350:i32, "request number OUT"=w3349:i32, "bytes per pixel OUT"=w3346:i32)  [unwired: 13 out]
            n2299 = call "DMR_GetImageRequestBufferImageData.vi"("driver handle IN"=w3350, "request number IN"=w3349, "bytes per pixel IN"=w3346, "X-offset IN"=w3345, "Y-offset IN"=w3345, "height IN"=w3343, "width IN"=w3344) -> ("driver handle OUT"=w3348:u32, "request number OUT"=w3347:u32, "image OUT"=w3340:u32[][])  [unwired: 10 out]
            n2300 = call "DMR_ImageRequestUnlock.vi"("request number IN"=w3347, "driver handle IN"=w3348) -> ("driver handle OUT"=w3353:i32)  [unwired: 1 in, 2 out]
            n2301 = case shown="True" "Averaging" {
              tunnel: w3340 -> [w3396 w3401]
              tunnel: [w3396 w3400] -> w3336
              tunnel: w3339 -> [_ w3398]
              frame False {
              }
              frame True {
                (unwired) 1
                w3406 = 1
                n2302 = feedback #2(w3398) -> (w3397:u32[][])
                n2303 = Add(x=w3401, y=w3397) -> (x+y=w3402:u32[][])
                n2304 = Select(t=w3398, s="Reset Averaging", f=w3402) -> (s? t:f=w3404:u32[][])
                n2305 = feedback-in #2(w3404) -> ()
                n2306 = feedback #3(w3406) -> (w3399:i32)
                n2307 = Divide(x=w3402, y=w3399) -> (x/y=w3403:dbl[][])
                n2308 = Increment(x=w3399) -> (x+1=w3407:i32)
                n2309 = To Unsigned Long Integer(number=w3403) -> (unsigned 32bit integer=w3400:u32[][])
                n2310 = Select(t=w3406, s="Reset Averaging", f=w3407) -> (s? t:f=w3405:i32)
                n2311 = feedback-in #3(w3405) -> ()
              }
            }
            n2312 = call "DMR_ImageRequestSingle.vi"("request control IN"=0, "driver handle IN"=w3353) -> ("driver handle OUT"=w3351:i32)  [unwired: 3 out]
            n2313 = disable-structure shown="Disabled" {
              disable-tunnel: w3336 -> [w3373 _]
              disable-tunnel: w3333 -> [w3372 _]
              frame Disabled {
                n2314 = To Double Precision Float(number=w3373) -> (double precision float=w3371:dbl[][])
                n2315 = In Range and Coerce(upper limit="Intensity Upper", x=w3371, lower limit="Intensity Lower") -> (coerced(x)=w3370:dbl[][])  [unwired: 1 out]
                n2316 = Subtract(x="Intensity Upper", y="Intensity Lower") -> (x-y=w3367:dbl)
                n2317 = Subtract(x=w3370, y="Intensity Lower") -> (x-y=w3368:dbl[][])
                n2318 = Divide(x=w3368, y=w3367) -> (x/y=w3369:dbl[][])
                n2319 = Multiply(x=255.0, y=w3369) -> (x*y=w3365:dbl[][])
                n2320 = To Unsigned Byte Integer(number=w3365) -> (unsigned 8bit integer=w3374:u8[][])
                n2321 = call "IMAQ ArrayToImage"("Image Pixels (U8)"=w3374, "Image"=w3372) -> ("Image Out"=w3361:T2)  [unwired: 4 in, 5 out]
                n2322 = First Call?() -> (First Call?: T/F=w3362:bool)
                n2323 = case shown="True" w3362 {
                  tunnel: w3361 -> [w3375 w3386]
                  frame False {
                    n2324 = flat-sequence {
                      tunnel: w3375 -> [w3381]
                      frame #0 {
                        w3378 = FALSE ("Get/Set Status? (Set)")
                        w3377 = 0 ("Window Number (0...15)")
                        n2325 = call "IMAQ WindSize"("Get/Set Status? (Set)"=w3378, "Window Number"=w3377) -> ("Width & Height out"=→"Window Size":cluster{"Width":i32, "Height":i32})  [unwired: 4 in, 2 out]
                        n2326 = call "IMAQ WindMove"("Window Number (0...15)"=w3377, "Get/Set Status? (Set)"=w3378) -> ("Coordinates (screen)"=→"Window Position":cluster{"X Position":i32, "Y Position":i32})  [unwired: 3 in, 1 out]
                        n2327 = call "IMAQ WindDraw"("Resize to Image Size? (Y)"=FALSE, "Window Number (0...15)"=w3377, "Image"=w3381) -> ()  [unwired: 7 in, 2 out]
                      }
                      frame #1 {
                        n2328 = call "IMAQ WindZoom 2"("Center Point"="Center Point", "Zoom to Fit? (False)"=FALSE, "Zoom Factor"="Zoom Factor") -> ()  [unwired: 5 in, 4 out]
                      }
                    }
                  }
                  frame True {
                    n2329 = flat-sequence {
                      tunnel: w3386 -> [w3389]
                      tunnel: [w3387] -> w3385
                      tunnel: w3385 -> [w3391]
                      frame #0 {
                        w3388 = TRUE ("Resize to Image Size? (Y)")
                        w3387 = 0 ("Window Number (0...15)")
                        n2330 = call "IMAQ WindNonTearing"("Window Number"=w3387, "NonTearing? (True)"=w3388) -> ()  [unwired: 8 in, 2 out]
                        n2331 = call "IMAQ WindDraw"("Resize to Image Size? (Y)"=w3388, "Window Number (0...15)"=w3387, "Image"=w3389) -> ()  [unwired: 7 in, 2 out]
                      }
                      frame #1 {
                        n2332 = call "IMAQ WindSize"("Scrollbars? (N)"=FALSE, "Width & Height"="Initial Window Size", "Window Number"=w3391) -> ()  [unwired: 3 in, 3 out]
                        n2333 = call "IMAQ WindMove"("Window Number (0...15)"=w3391, "Coordinates (screen)"="Initial Window Position") -> ()  [unwired: 3 in, 2 out]
                      }
                    }
                  }
                }
              }
              frame Enabled {
              }
            }
            n2334 = To Unsigned Byte Integer(number=w3336) -> (unsigned 8bit integer=w3335:u8[][])
            n2335 = call "IMAQ ArrayToImage"("Image Pixels (U8)"=w3335, "Image"=w3332) -> ("Image Out"=w3330:T2)  [unwired: 4 in, 5 out]
            n2336 = case shown="True" "Save Video" {
              tunnel: w3337 -> [_ w3395]
              tunnel: w3330 -> [_ w3394]
              frame False {
              }
              frame True {
                n2337 = call "IMAQ AVI Write Frame"("Image"=w3394, "Avi Refnum"=w3395) -> ()  [unwired: 2 in, 8 out]
              }
            }
            n2338 = case shown="True" "Save Image" {
              tunnel: w3335 -> [_ w3410]
              tunnel: w3334 -> [_ w3409]
              frame False {
              }
              frame True {
                n2339 = call <vilib>:"Flatten Pixmap.vi"("colors"=w3409, "8-bit pixmap"=w3410) -> ("image data"=w3416:T34)  [unwired: 4 in, 5 out]
                n2340 = call "Create new save file.vi"("Insert"="video_frame_" ("string"), "Ext"=".bmp" ("string"), "Index In"="Image Index") -> ("Path Out"=w3412:path, "Index Out"=w3417:dbl)
                n2341 = Increment(x=w3417) -> (x+1=w3411:dbl)
                n2342 = local write "Image Index"(w3411) -> ()
                n2343 = call <vilib>:"Write BMP File.vi"("image data"=w3416, "path to BMP file"=w3412) -> ()  [unwired: 1 in, 9 out]
              }
            }
            n2344 = case shown="True" "Target" {
              tunnel: w3330 -> [w3356 w3360]
              tunnel: [w3356 w3358] -> w3329
              frame False {
              }
              frame True {
                n2345 = local read "Target coordinates"() -> (w3357:cluster{"X1":dbl, "Y1":dbl, "X2":dbl, "Y2":dbl})
                n2346 = call "IMAQ Overlay Oval"("Color"=u32 16711680, "Bounding Rectangle"=w3357, "Image"=w3360) -> ("Image Out"=w3358:T2)  [unwired: 7 in, 1 out]
              }
            }
            "Primary Video Display" <- w3329
          }
        }
        n2347 = node-c288(w3291) -> ()  [unwired: 1 out]
      }
      n2348 = node-c288(w3275) -> ()  [unwired: 1 out]
      n2349 = call "DMR_CloseDevice2.vi"("driver handle IN"=w3280) -> ()  [unwired: 1 in, 4 out]
    }
    frame #4 {
      n2350 = call "DMR_Close.vi"() -> ()  [unwired: 1 out]
    }
  }
  n2351 = local write "Offset (nm)"(0.0 ("Offset (nm)")) -> ()
  n2352 = local write "Bead Mean (nm)"(0.0 ("Bead Mean (nm)")) -> ()
  n2353 = local write "Total Volume\nFlowed P1 (uL)"(w12) -> ()
  n2354 = local write "Total Volume\nFlowed Samp (uL)"(w12) -> ()
  n2355 = local write "Total Volume\nFlowed P3 (uL)"(w12) -> ()
  n2356 = node-c288(i64 1 ("Period"), 1 ("Processor")) -> (w191:T21)  [unwired: 2 out]
  n2357 = timed-loop "Acquire Data" {
    tunnel: w18 -> [w3725]
    tunnel: w67 -> [w3724]
    tunnel: [w3754] -> w284
    tunnel: [w3749] -> w282
    timing: w191 -> [_]
    timing-out: [_] -> w190
    tunnel: w86 -> [w3563]
    stop <- "Stop All" stop-if-true
    w3481 = "Initialize"
    w3550 = "NI_ChannelName" ("name")
    n2358 = node-c288() -> ()  [unwired: 2 out]
    n2359 = First Call?() -> (First Call?: T/F=w3516:bool)
    n2360 = Or(x="Reset", y=w3516) -> (x .or. y?=w3517:bool)
    n2361 = local read "Flushing P1"() -> (w3436:bool)
    n2362 = case "Reset data stream" shown="True" w3517 {
      tunnel: w3725 -> [w4792 w4800]
      tunnel: w3724 -> [w4791 w4799]
      tunnel: [w4792 w4794] -> w3429
      tunnel: [w4791 w4793] -> w3720
      frame False {
      }
      frame True {
        w4797 = TRUE ("AI to FIFO")
        n2363 = local write "Overflow (data lost)"(FALSE ("Overflow (data lost)")) -> ()
